vi "event_structure_with_global.vi"() -> ()   [LabVIEW 2023]
uses:
  Global 1.vi
panel:
  out "Array 2":bool[](array[boolean])
  in  "check":bool
  in  "stop":bool
  out "Array":bool[](array[boolean])
  in  "Enum":enum16{"XOr", "Or", "And"}(ring)
  out "Boolean 24":bool
  out "Boolean 23":bool
  out "Boolean 22":bool
  out "Boolean 21":bool
  out "Boolean 20":bool
  out "Boolean 19":bool
  out "Boolean 18":bool
  out "Boolean 17":bool
  in  "Boolean 16":bool
  in  "Boolean 15":bool
  in  "Boolean 14":bool
  in  "Boolean 13":bool
  in  "Boolean 12":bool
  in  "Boolean 11":bool
  in  "Boolean 10":bool
  in  "Boolean 9":bool
  in  "Boolean 8":bool
  in  "Boolean 7":bool
  in  "Boolean 6":bool
  in  "Boolean 5":bool
  in  "Boolean 4":bool
  in  "Boolean 3":bool
  in  "Boolean 2":bool
  in  "Boolean":bool
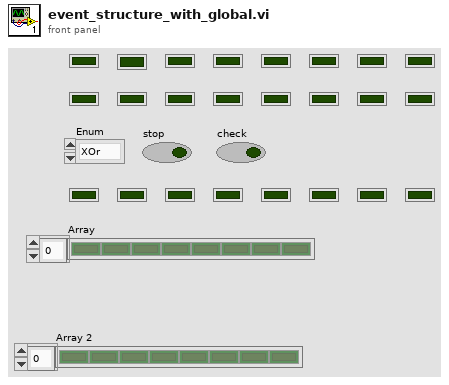
[diagram p1: front panel]
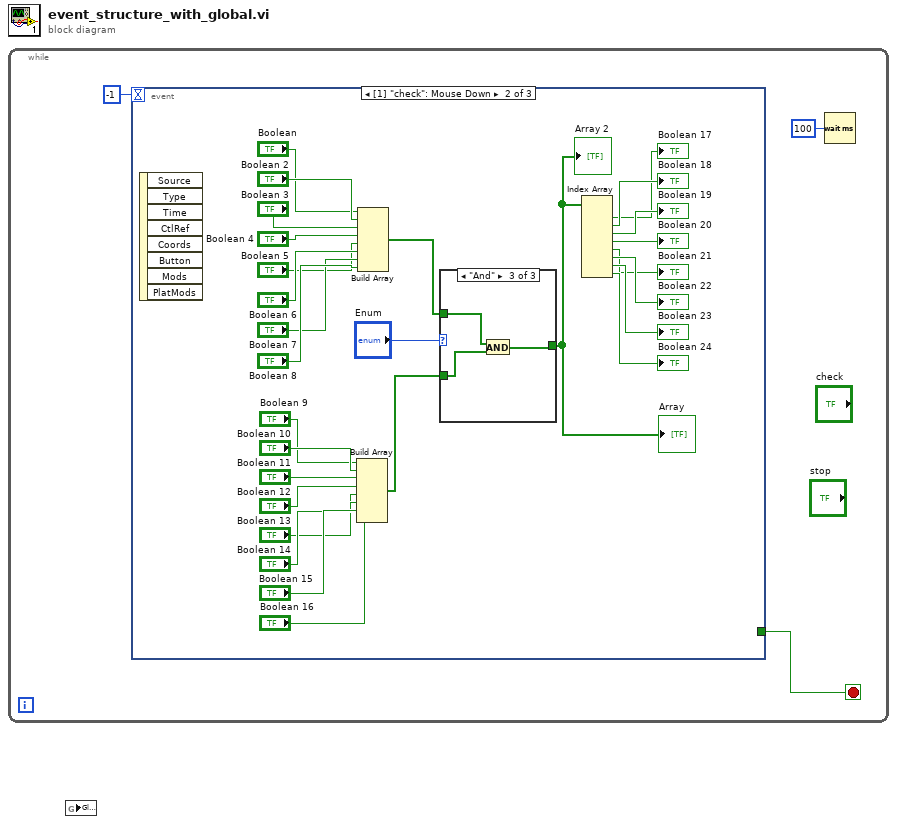
[diagram p0: block diagram]
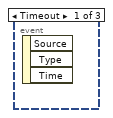
[diagram p2: hidden frame]
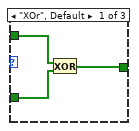
[diagram p3: hidden frame]
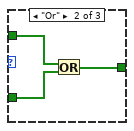
[diagram p4: hidden frame]
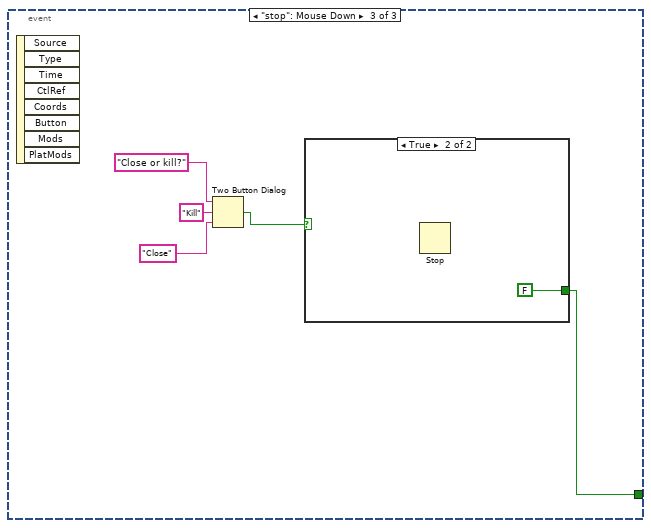
[diagram p5: hidden frame]
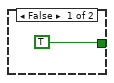
[diagram p6: hidden frame]
diagram:
  n1 = while {
    stop <- w2 stop-if-true
    n2 = event shown="[1] \"check\": Mouse Down" {
      selector: _ -> [_ _ _]
      dyn-events: _ -> [_ _ _]
      timeout: -1 -> [_ _ _]
      tunnel: [_ _ w41] -> w2
      event Timeout {
        n3 = event-data() -> ()  [unwired: 1 in, 3 out]
      }
      event "check": Mouse Down {
        n4 = event-data() -> ()  [unwired: 1 in, 8 out]
        n5 = Build Array("Boolean 9", "Boolean 10", "Boolean 11", "Boolean 12", "Boolean 13", "Boolean 14", "Boolean 15", "Boolean 16") -> (w22:bool[])
        n6 = Build Array("Boolean", "Boolean 2", "Boolean 3", "Boolean 4", "Boolean 5", "Boolean 6", "Boolean 7", "Boolean 8") -> (w21:bool[])
        n7 = case shown="\"And\"" "Enum" {
          tunnel: w21 -> [w32 w36 w39]
          tunnel: w22 -> [w33 w37 w40]
          tunnel: [w34 w35 w38] -> w23
          frame "XOr", Default {
            n8 = Exclusive Or(1:w33, 2:w32) -> (0:w34:bool[])
          }
          frame "Or" {
            n9 = Or(x=w36, y=w37) -> (x .or. y?=w35:bool[])
          }
          frame "And" {
            n10 = And(x=w39, y=w40) -> (x .and. y?=w38:bool[])
          }
        }
        "Array" <- w23
        "Array 2" <- w23
        n11 = Index Array(array=w23) -> (element #1=→"Boolean 17":bool, element #2=→"Boolean 18":bool, element #3=→"Boolean 19":bool, element #4=→"Boolean 20":bool, element #5=→"Boolean 21":bool, element #6=→"Boolean 22":bool, element #7=→"Boolean 23":bool, element #8=→"Boolean 24":bool)  [unwired: 8 in]
      }
      event "stop": Mouse Down {
        n12 = event-data() -> ()  [unwired: 1 in, 8 out]
        n13 = Two Button Dialog(message="Close or kill?", 1:"Close" ("F button name (\"Cancel\")"), 2:"Kill" ("T button name (\"OK\")")) -> (T button?=w45:bool)
        n14 = case shown="True" w45 {
          tunnel: [TRUE FALSE] -> w41
          frame False {
          }
          frame True {
            n15 = Stop() -> ()  [unwired: 1 in]
          }
        }
      }
    }
    n16 = Wait (ms)(milliseconds to wait=u32 100) -> ()  [unwired: 1 out]
  }
  n17 = global read "Global 1.vi" item#-1() -> ()  [unwired: 1 in]
